vi "Get Channel Coupling Supported.vi"(8 "error in (no error)":errorcluster, 11 "board_handle":u8) -> (0 "error out":errorcluster, 2 "Is supported":bool, 3 "board_handle out":u8)   [LabVIEW 2024, in "AIM ARINC 429 Hardware API.lvlib"]
doc: "AI_LIB_FUNC AiReturn AI_CALL_CONV Api429BoardChannelCouplingIsSupported( AiUInt8 board_handle, AiBoolean* is_supported );"
uses:
  AIM ARINC 429 Hardware API.lvlib
  <instrlib>/AIM GmbH/_ARINC-429/VIs/Library/Api429Lib Error Desc Get.vi
  <instrlib>/AIM GmbH/_ARINC-429/subvi/Get Error Number Offset.vi
  <vilib>/Utility/error.llb/Error Cluster From Error Code.vi
  <instrlib>/AIM GmbH/_ARINC-429/AIM429LV.lvlib
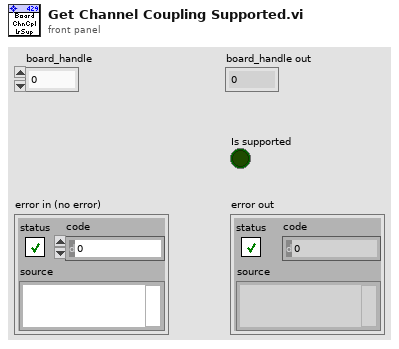
[diagram p1: front panel]
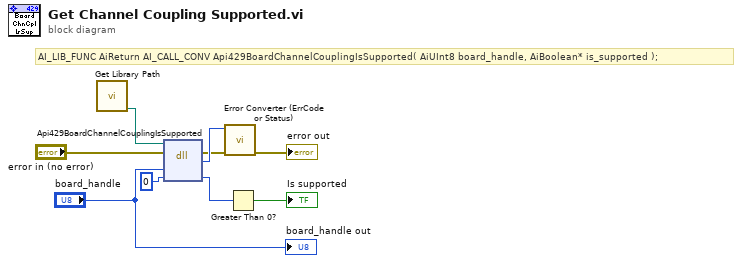
[diagram p0: block diagram]
diagram:
  # "AI_LIB_FUNC AiReturn AI_CALL_CONV Api429BoardChannelCouplingIsSupported( AiUInt8 board_handle, AiBoolean* is_supported );"
  n1 = call <instrlib>:"Get Library Path.vi"() -> ("GlobalDLLPath"=w4:path)  [unwired: 11 in]
  n2 = dll-call lib="?" fn="Api429BoardChannelCouplingIsSupported"(path in=w4, error in="error in (no error)", "board_handle"="board_handle", "pucResult"=u8 0) -> (error out=w6:errorcluster, "return type"=w9:i32, "pucResult"=w2:u8)  [unwired: 2 in, 1 out]
  n3 = call <instrlib>:"Error Converter (ErrCode or Status).vi"("error in (no error)"=w6, "error code"=w9) -> ("error out"=→"error out":errorcluster)  [unwired: 9 in]
  n4 = Greater Than 0?(x=w2) -> (x > 0?=→"Is supported":bool)
  "board_handle out" <- "board_handle"
